vi "Vector_Norm.vi"(11 "Input Vector":T1) -> (3 "norm":dbl)   [LabVIEW 2019, in "Trajectory_Library.lvlib"]
doc: "Calculate the dot product of two vectors\n\nInputs:\n -- InputVector 1 -- Input vector 1\n -- InputVector 2 -- Input vector 2. This vector must have at least as many rows as vector 1.\n\nOutputs:\n -- Dot Product -- Calculated vector dot product."
uses:
  <vilib>/Analysis/Matrix/Datatypes/RealMatrix.ctl
  Trajectory_Library.lvlib
  <vilib>/Analysis/Matrix/NI_Matrix.lvlib
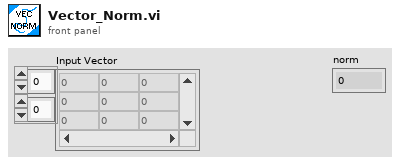
[diagram p1: front panel]
types:
  T1 = typedef "NI_Matrix.lvlib/RealMatrix.ctl" = dbl[][]
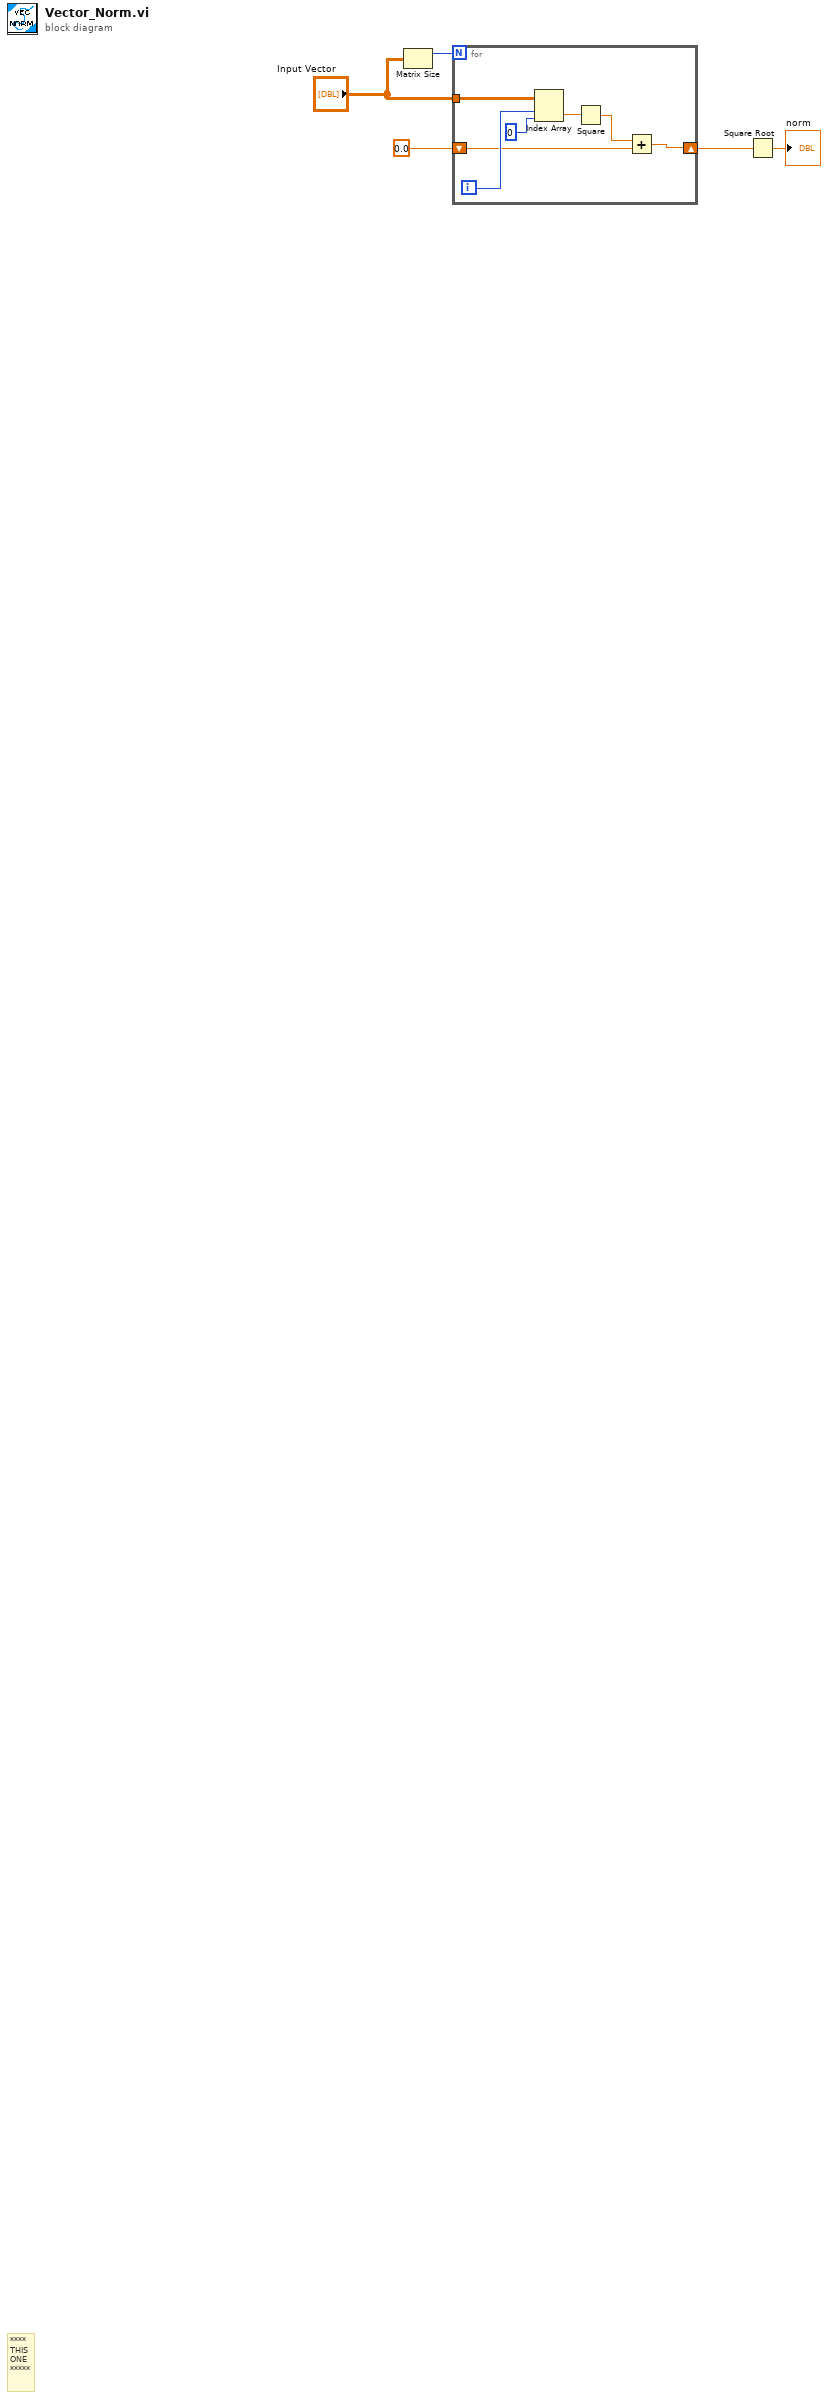
[diagram p0: block diagram]
diagram:
  # "****\nTHIS\nONE\n*****"
  n1 = Matrix Size(0:"Input Vector") -> (1:w5:i32)  [unwired: 1 out]
  n2 = for {
    N: w5 -> [_]
    tunnel: "Input Vector" -> [w10]
    shift-right: [w6] -> w2
    shift-left: 0.0 -> [w7]
    i -> [w12]
    n3 = Index Array(array=w10, index (row)=w12, index (col)=0) -> (element=w9:dbl)
    n4 = Square(x=w9) -> (x^2=w8:dbl)
    n5 = Add(x=w8, y=w7) -> (x+y=w6:dbl)
  }
  n6 = Square Root(x=w2) -> (sqrt(x)=→"norm":dbl)
